vi "AgPSA _Single Sweep and Peak Search.vi"(6 "Cal Route":string[](array[string])=["", "", ""], 7 "Cal?":bool, 8 "error in (no error)":errorcluster, 9 "Center (Hz)":dbl, 10 "Span (Hz)":dbl, 11 "VISA Refnum in":refnum<visa-resource-name>) -> (0 "error out":errorcluster, 1 "Calibrated Marker Amplitude":dbl, 2 "Marker Position":dbl, 3 "VISA Refnum out":refnum<visa-resource-name>)   [LabVIEW 2015]
uses:
  <instrlib>/Agilent ESA PSA Series/Agilent ESA PSA Series.lvlib
panel:
  in  "Active Marker":u16(ring)=1 items=["Marker1"=1, "Marker2"=2, "Marker3"=3, "Marker4"=4]
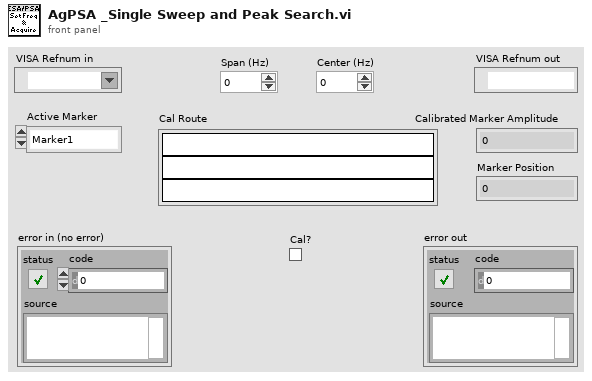
[diagram p1: front panel]
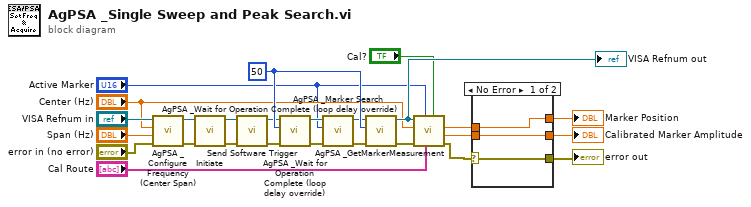
[diagram p0: block diagram]
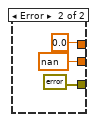
[diagram p2: hidden frame]
diagram:
  w26 = u32 50 ("loop delay (ms)")
  n1 = call "AgPSA _Configure Frequency (Center Span).vi"("error in (no error)"="error in (no error)", "Span (2 GHz)"="Span (Hz)", "Center Frequency (2 GHz)"="Center (Hz)", "VISA resource name"="VISA Refnum in") -> ("error out"=w19:errorcluster, "VISA resource name out"=w18:refnum<visa-resource-name>)  [unwired: 6 in]
  n2 = call <instrlib>:"Initiate.vi"("error in (no error)"=w19, "VISA resource name"=w18) -> ("error out"=w17:errorcluster, "VISA resource name out"=w16:refnum<visa-resource-name>)  [unwired: 8 in]
  n3 = call <instrlib>:"Send Software Trigger.vi"("error in (no error)"=w17, "VISA resource name"=w16) -> ("error out"=w21:errorcluster, "VISA resource name out"=w20:refnum<visa-resource-name>)  [unwired: 8 in]
  n4 = call "AgPSA _Wait for Operation Complete (loop delay override).vi"("error in (no error)"=w21, "loop delay (ms)"=w26, "VISA resource name"=w20) -> ("error out"=w23:errorcluster, "VISA resource name out"=w22:refnum<visa-resource-name>)  [unwired: 7 in]
  n5 = call "AgPSA _Marker Search.vi"("error in (no error)"=w23, "Active Marker"="Active Marker", "VISA resource name"=w22) -> ("error out"=w25:errorcluster, "VISA resource name out"=w24:refnum<visa-resource-name>)  [unwired: 7 in]
  n6 = call "AgPSA _Wait for Operation Complete (loop delay override).vi"("error in (no error)"=w25, "loop delay (ms)"=w26, "VISA resource name"=w24) -> ("error out"=w10:errorcluster, "VISA resource name out"=w12:refnum<visa-resource-name>)  [unwired: 7 in]
  "VISA Refnum out" <- w12
  n7 = call "AgPSA _GetMarkerMeasurement.vi"("Cal?"="Cal?", "Cal Route"="Cal Route", "Active Marker (1: Marker1)"="Active Marker", "error in (no error)"=w10, "Cal Freq (Hz)"="Center (Hz)", "PSA In"=w12) -> ("error out"=w6:errorcluster, "Calibrated Marker Amplitude"=w3:dbl, "Marker Position"=w1:dbl)  [unwired: 2 in, 1 out]
  n8 = case shown="No Error" w6 {
    selector: w6 -> [w29 _]
    tunnel: [w29 errorcluster {"status"=FALSE, "code"=0, "source"=""} ("error constant")] -> w5
    tunnel: [w28 nan ("Calibrated Marker Amplitude")] -> w4
    tunnel: w3 -> [w28 _]
    tunnel: [w27 0.0 ("Marker Position")] -> w2
    tunnel: w1 -> [w27 _]
    frame No Error {
    }
    frame Error {
    }
  }
  "error out" <- w5
  "Calibrated Marker Amplitude" <- w4
  "Marker Position" <- w2
